vi "Global Tube Length.vi"() -> ()   [LabVIEW 2019]
panel:
  in  "Tube Lengths":dbl[](array[numeric]) format="%.3f"
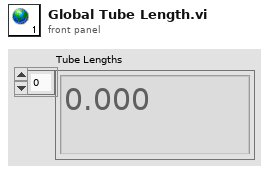
[diagram p1: front panel]
diagram:
